vi "File.vi"() -> ()   [LabVIEW 2017]
panel:
  in  "Folder Path":path=path "C:/Projects/builds/Kinetics/Kinetics/Release"
  in  "base path":path=path "C:/Projects/builds/Kinetics/Kinetics/Release"
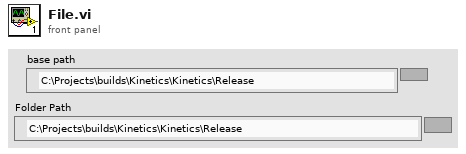
[diagram p1: front panel]
types:
  T1 = enum16{"open", "replace", "create", "open or create", "replace or create", "replace or create with confirmation"}
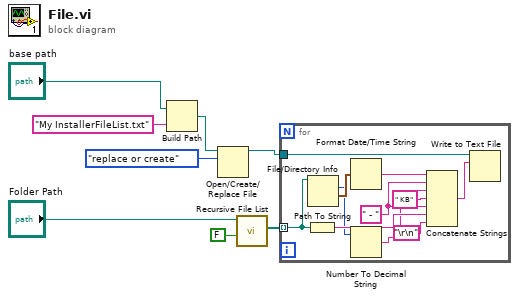
[diagram p0: block diagram]
diagram:
  n1 = Build Path(base path="base path", name or relative path="My InstallerFileList.txt") -> (appended path=w5:path)
  n2 = Open/Create/Replace File(file path (use dialog)=w5, operation (0:open)=T1."replace or create") -> (refnum out=w2:refnum<file>)  [unwired: 4 in, 2 out]
  n3 = call <vilib>:"Recursive File List.vi"("Continue Recursing on Error? (F)"=FALSE, "Folder Path"="Folder Path") -> ("All Files in Dir"=w6:path[])  [unwired: 5 in, 4 out]
  n4 = for {
    tunnel: w6 -> [w15] mode=indexing
    tunnel: w2 -> [w18]
    w12 = " - " ("string")
    n5 = Path To String(path=w15) -> (string=w19:string)
    n6 = File/Directory Info(path=w15) -> (size=w11:i64, last mod=w14:timestamp)  [unwired: 1 in, 5 out]
    n7 = Format Date/Time String(seconds (now)=w14) -> (date/time string=w13:string)  [unwired: 2 in]
    n8 = Number To Decimal String(number=w11) -> (decimal integer string=w10:string)  [unwired: 1 in]
    n9 = Concatenate Strings(w13, w12, w10, " KB" ("string"), w12, w19, "\r\n") -> (w17:string)
    n10 = Write to Text File(file (use dialog)=w18, text=w17) -> ()  [unwired: 2 in, 3 out]
  }
